vi "KepcoBOP Configure External Refernces .vi"(0 "VISA Session":refnum<visa-resource-name>, 5 "Model In":string, 7 "Mode (Fixed)":T1(ring), 9 "Limit mode":enum16{"Fixed", "External", "Lesser"}(ring), 11 "error in (no error)":errorcluster {"code" format="%.0x"}) -> (4 "VISA Session Out":refnum<visa-resource-name>, 6 "Model Out":string, 15 "error out":errorcluster {"code" format="%.0x"})   [LabVIEW 2010]
doc: "Configures External references to control Main channel and Limits."
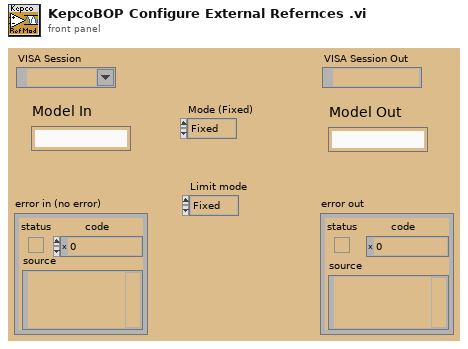
[diagram p1: front panel]
types:
  T1 = enum16{"Fixed", "List", "Transient", "External", "Gain", "Protect", "Additive"}
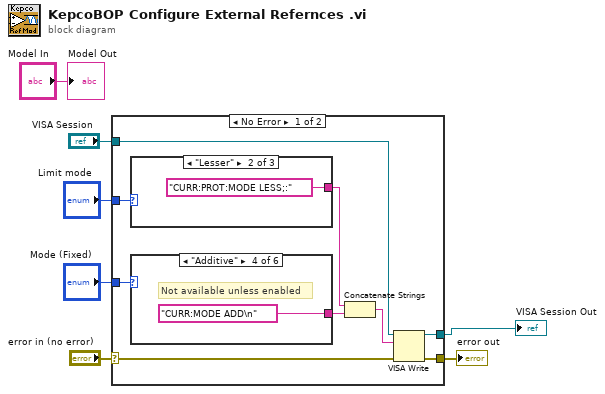
[diagram p0: block diagram]
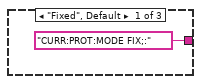
[diagram p2: hidden frame]
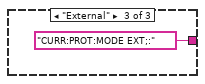
[diagram p3: hidden frame]
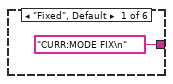
[diagram p4: hidden frame]
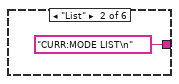
[diagram p5: hidden frame]
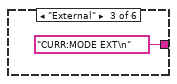
[diagram p6: hidden frame]
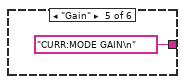
[diagram p7: hidden frame]
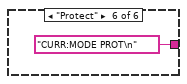
[diagram p8: hidden frame]
diagram:
  n1 = case shown="No Error" "error in (no error)" {
    selector: "error in (no error)" -> [w15 w26]
    tunnel: "VISA Session" -> [w16 w27]
    tunnel: [w14 w26] -> w5
    tunnel: [w13 w27] -> w4
    tunnel: "Mode (Fixed)" -> [w12 _]
    tunnel: "Limit mode" -> [w11 _]
    frame No Error {
      n2 = case shown="\"Lesser\"" w11 {
        tunnel: ["CURR:PROT:MODE FIX;:" "CURR:PROT:MODE LESS;:" "CURR:PROT:MODE EXT;:"] -> w10
        frame "Fixed", Default {
        }
        frame "Lesser" {
        }
        frame "External" {
        }
      }
      n3 = case shown="\"Additive\"" w12 {
        tunnel: ["CURR:MODE FIX\n" "CURR:MODE LIST\n" "CURR:MODE EXT\n" "CURR:MODE ADD\n" "CURR:MODE GAIN\n" "CURR:MODE PROT\n"] -> w9
        frame "Fixed", Default {
        }
        frame "List" {
        }
        frame "External" {
        }
        frame "Additive" {
          # "Not available unless enabled"
        }
        frame "Gain" {
        }
        frame "Protect" {
        }
      }
      n4 = Concatenate Strings(w10, w9) -> (w8:string)
      n5 = VISA Write(VISA resource name=w16, write buffer=w8, error in (no error)=w15) -> (VISA resource name out=w13:refnum<visa-resource-name>, error out=w14:errorcluster)  [unwired: 1 out]
    }
    frame Error {
    }
  }
  "error out" <- w5
  "VISA Session Out" <- w4
  "Model Out" <- "Model In"
